vi "LSCI332ScanCalibName.vi"(0 "VISA Rsrc":refnum<visa-resource-name>="GPIB0::12::INSTR" caption="Adresse du contrôlleur", 11 "error in":errorcluster) -> (6 "Courbe Calib":string[][](table) caption="Courbes de Calibration", 15 "error out":errorcluster)   [LabVIEW 2019]
doc: "Ce Vi écrit l'entête et les points d'une courbe de calibration dans l'emplacement spécifié du contrôlleur de température"
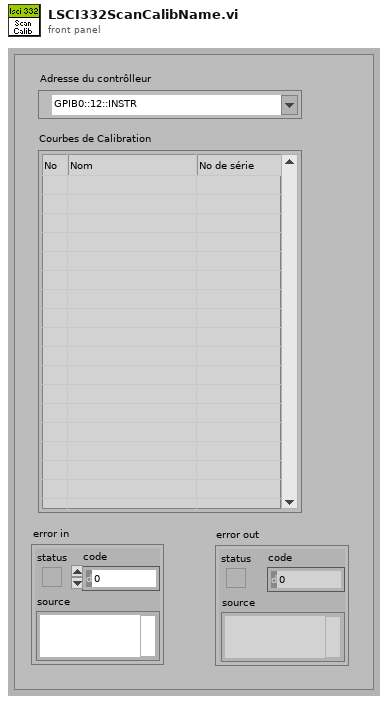
[diagram p1: front panel]
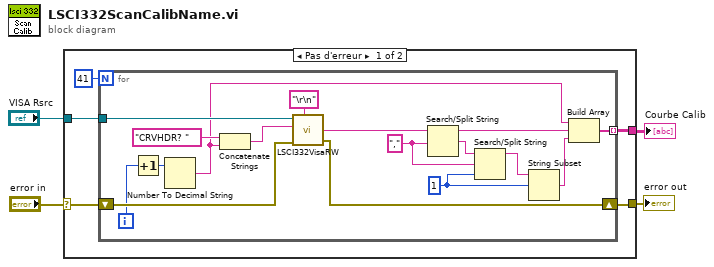
[diagram p0: block diagram]
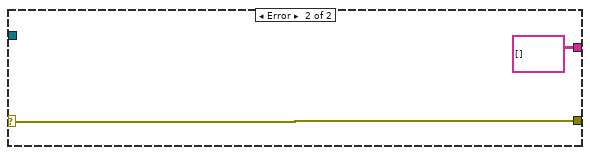
[diagram p2: hidden frame]
diagram:
  n1 = case shown="Pas d'erreur" "error in" {
    selector: "error in" -> [w7 w28]
    tunnel: "VISA Rsrc" -> [w8 _]
    tunnel: [w6 w28] -> w2
    tunnel: [w5 string[][] []] -> w1
    frame No Error {
      n2 = for {
        N: 41 -> [_]
        tunnel: w8 -> [w26]
        shift-right: [w24] -> w6
        shift-left: w7 -> [w25]
        tunnel: [w15] -> w5 mode=indexing
        i -> [w22]
        w11 = 1
        w17 = ","
        n3 = Increment(x=w22) -> (x+1=w21:i32)
        n4 = Number To Decimal String(number=w21) -> (decimal integer string=w10:string)  [unwired: 1 in]
        n5 = Concatenate Strings("CRVHDR? ", w10) -> (w12:string)
        n6 = call <userlib>:"LSCI332VisaRW.vi"("error in (no error)"=w25, "EOS (Aucun)"="\r\n", "ChaineCom"=w12, "VISA Rsrc"=w26) -> ("error out"=w24:errorcluster, "ChaineRep"=w19:string)  [unwired: 3 in, 2 out]
        n7 = Search/Split String(string=w19, search string/char (-)=w17) -> (substring before match=w16:string, match + rest of string=w18:string)  [unwired: 1 in, 1 out]
        n8 = Search/Split String(string=w18, search string/char (-)=w17, offset (0)=w11) -> (substring before match=w14:string)  [unwired: 2 out]
        n9 = String Subset(string=w14, offset (0)=w11) -> (substring=w13:string)  [unwired: 1 in]
        n10 = Build Array(w10, w16, w13) -> (w15:string[])
      }
    }
    frame Error {
    }
  }
  "error out" <- w2
  "Courbe Calib" <- w1
